vi "SPI_GetMode.vi"(5 "Device":i32, 7 "Bus":i32=1, 8 "error in":errorcluster) -> (0 "error out":errorcluster, 4 "Mode":u8 format="%02b")   [LabVIEW 2014, in "GPIO.lvlib"]
doc: "Get the SPI mode for the current device. Mode is a two-bit value (0-3), the MSB determines the clock polarity and the LSB determines the phase."
uses:
  GPIO.lvlib
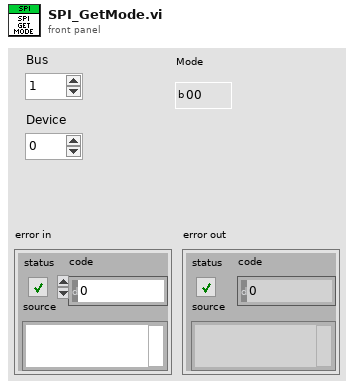
[diagram p1: front panel]
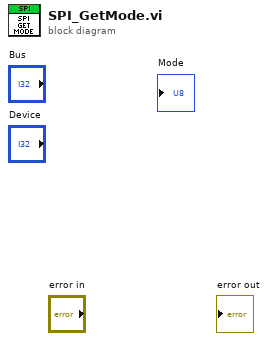
[diagram p0: block diagram]
diagram:
